vi "main.vi"(0 "Test Pins":T7, 1 "Caller Information":T8, 5 "Test Inputs":T12={"Input Voltage in V"=6.0, "Load Current in A"=[], "Nominal Output Voltage in V"=0.0, "Advance Setting"={"Prepare"={"Load SMU Output Function"=enum."VoltageSource"}, "Stimulus And Measure"={"Loop Delay in milliSecond"=1}}}, 11 "error in":errorcluster) -> (4 "Test Results":T11 {"Load Regulation in mV/mA" format="%#.5g"; "Measured Input Voltage in V" format="%#.5g"; "Measured Input Current in A" format="%#.5g"; "Measured Load Current in A" format="%#.5g"; "Measured Output Voltage in V" format="%#.5g"}, 15 "error out":errorcluster)   [LabVIEW 2020, in "LDO Load Regulation.lvlib"]
doc: "<b>Caller</b> Information is input for framework components. Mode should be set to <b>Automation</b> when running from TestStand. Sequence Context should be set to <b>ThisContext</b> when running from TestStand. The values will be updated everytime the setting is applied using \"Edit\" dialog.\n\n<b>Test Pins</b> is names of pins available in the pinmap file. Provide the right pins for the required functionality.\n\n<b>Test Inputs</b> is input required for the measurement to perform.\n\n<b>error in</b> is meant for the sequencing. <b>error in</b> should be <b>no error</b> always.\n\n<b>Test Results</b> contains all the measured data during the measurement and processed results.\n\n<b>error out</b> contains the error occured during measurement.\n\nCheck measurement documentation for more information (<Program Files>\\Soliton Technologies\\MeasurementSuite\\CodeModules\\LDO\\LDO Load Regulation.pdf)"
uses:
  LDO Load Regulation.lvlib
  Typedefs/Test Results.ctl
  Typedefs/Test Inputs.ctl
  Typedefs/Advance Settings.ctl
  Typedefs/Adv Setup.ctl
  Reusables/Instrument APIs/Load Output Function.ctl
  Typedefs/Adv StimulusMeasure.ctl
  <userlib>/_Soliton/Measurement Suite/Reusables/Plugin Common/Typedefs/Caller Events.ctl
  <userlib>/_Soliton/Measurement Suite/Reusables/Plugin Common/Typedefs/Caller Information.ctl
  <userlib>/_Soliton/Measurement Suite/Reusables/Plugin Common/Typedefs/Caller Mode.ctl
  Typedefs/Test Pins.ctl
  Typedefs/Pin Dropdown.ctl
  <userlib>/_Soliton/Measurement Suite/Reusables/Plugin Common/Typedefs/Termination Monitor Info.ctl
  <vilib>/Utility/error.llb/DialogType.ctl
  dc46d5cc-eb00-4f7e-b59b-e7fbb9f2ed4c.vi
  f0cc231b-6294-4813-9d5b-a7ddc5043ff2.vi
  f8cfc4b9-01f6-4b8f-8ca0-5ef2fe22dc8a.vi
  be024a05-4f6c-4aec-bf2b-5f4e194505bf.vi
  d9360132-6dee-4b9e-876e-39170c807331.vi
  f5d431a0-41a8-4d91-8ed4-f3030fcb2f72.vi
  a0f7aff6-54e5-4632-b7fd-dab2f19ee789.vi
  9bf00ac7-c58e-45e8-95f2-565a27dd0209.vi
  d12a1fd7-5478-4f09-8baf-cc2a5bf82fd5.vi
  97045b22-c088-492e-b8fe-756b4ca626c0.vi
  c2b1c575-6273-4f01-9f2a-bc195d2502fa.vi
  <userlib>/_Soliton/Measurement Suite/Reusables/InstrumentSessionAPIs/SessionManagerApiPath.vi
  <vilib>/Utility/sysdir.llb/Get System Directory.vi
  <vilib>/Utility/LVLibp/Get Exported File Path.vi
  <userlib>/_Soliton/Measurement Suite/Reusables/Errors/Error 6001.vi
  <userlib>/_Soliton/Measurement Suite/Reusables/Plugin Common/Plugin Common.lvlib
  <userlib>/_Soliton/Measurement Suite/Reusables/Queue Driver/Plugin Queue Driver.lvlib
panel:
  out "Progress":i32(slide) scale=-1.0..5.0
  in  "Terminate":bool
  in  "Run":bool caption="Measure"
  in  "Exit":bool
  out "Header":string
  in  "Pages":T1(radio)
  out "Tab Control":T2(tab)
  in  "SystemSetup":T4={"Set Input Voltage"={"PinStatus"=0, "PinName"="", "Info"=TRUE}, "Measure Input Voltage"={"PinStatus"=0, "PinName"="", "Info"=TRUE}, "Measure Input Current"={"PinStatus"=0, "PinName"="", "Info"=TRUE}, "Set Load Current"={"PinStatus"=0, "PinName"="", "Info"=TRUE}, "Measure Output Voltage"={"PinStatus"=0, "PinName"="", "Info"=TRUE}, "Measure Load Current"={"PinStatus"=0, "PinName"="", "Info"=TRUE}}
  in  "Advanced Settings":bool
  in  "Input Voltage (V)":dbl=6.0 format="%#_6p"
  in  "Step Input":T5 {"Step Size (A)" min=0.0 format="%#_6p"; "Stop Value (A)" format="%#_6p"; "Start Value (A)" format="%#_6p"}
  in  "Customize Sweep Value":bool
  in  "Load Current (A)":dbl[](array[numeric]) format="%#_6p"
  in  "Nominal Output Voltage (V)":dbl format="%#_6p"
  in  "Customize Sweep Value":enum32{"Item 0", "Item 1"}(radio)
  out "Load Regulation (mV/mA)":dbl format="%#.3g"
  out "Result Tab":T6(tab)
  out "Line Regulation":cluster{"Iload (mA)":dbl[], "Vout (V)":dbl[]}(graph)
  out "Measured Values":string[][](table)
  out "Load Regulation (%)":dbl format="%#.3g"
  in  "Result Pages":T6(radio)
  in  "DataLogPath":path
  in  "Caller Events":T10
  in  "ErrorOccured":errorcluster
  # "Supports NIDmmInstrument"
  # "Supports NIDmmInstrument"
  # "Supports NIDCPowerInstrument"
  # "Supports NIDCPowerInstrument"
  # "Supports NIDCPowerInstrument"
  # "Supports NIDCPowerInstrument"
  # "Fill Load Current list using the following"
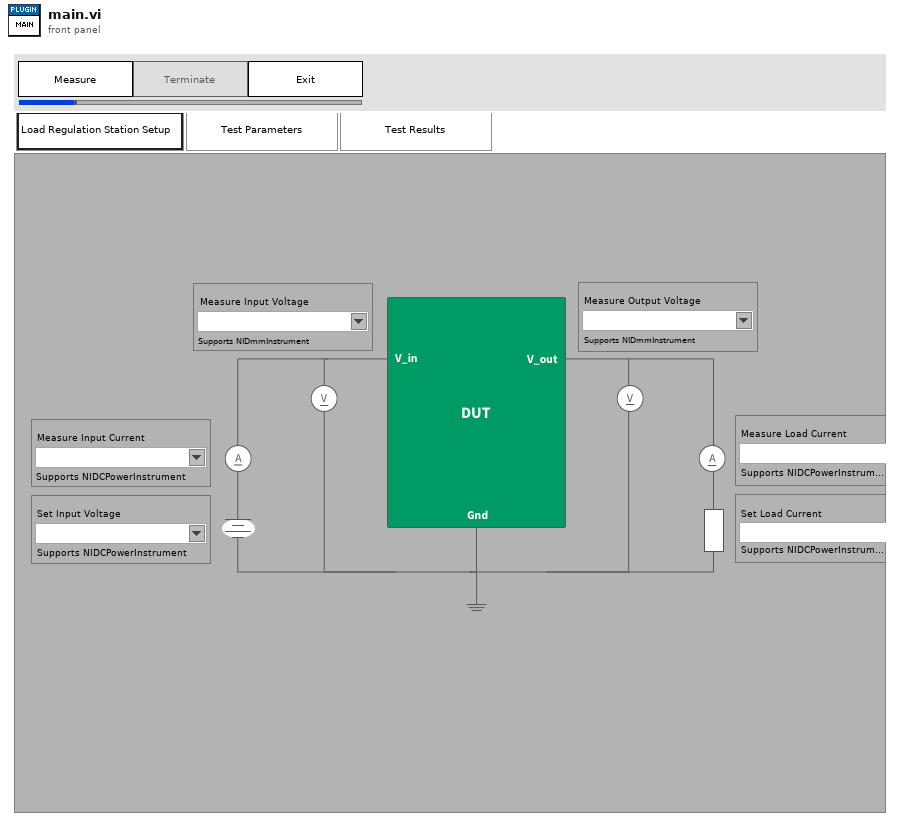
[diagram p1: front panel]
types:
  T1 = enum32{"Station Setup", "Test Parameters", "Test Results"}
  T2 = enum32{"Station Setup", "Test Parameters", "Test Results", "Debug"}
  T3 = typedef "LDO Load Regulation.lvlib/Pin Dropdown.ctl" = cluster{"PinStatus":u16, "PinName":string, "Info":bool}
  T4 = cluster{"Set Input Voltage":T3, "Measure Input Voltage":T3, "Measure Input Current":T3, "Set Load Current":T3, "Measure Output Voltage":T3, "Measure Load Current":T3}
  T5 = cluster{"Start Value (A)":dbl, "Stop Value (A)":dbl, "Step Size (A)":dbl}
  T6 = enum32{"Load Regulation Curve", "Measured Value Table View"}
  T7 = typedef "LDO Load Regulation.lvlib/Test Pins.ctl" = cluster{"Set Input Voltage":string, "Measure Input Voltage":string, "Measure Input Current":string, "Set Load Current":string, "Measure Output Voltage":string, "Measure Load Current":string}
  T8 = typedef "Plugin Common.lvlib/Caller Information.ctl" = cluster{"Mode":T9, "Sequence Context":refnum<k7>}
  T9 = typedef "Caller Mode.ctl" = enum16{"Standalone", "Automation", "MeasurementSuite"}
  T10 = typedef "Plugin Common.lvlib/Caller Events.ctl" = cluster{"Caller Event":refnum<user-event>}
  T11 = typedef "LDO Load Regulation.lvlib/Test Results.ctl" = cluster{"Measured Input Voltage in V":dbl[], "Measured Input Current in A":dbl[], "Measured Output Voltage in V":dbl[], "Measured Load Current in A":dbl[], "Load Regulation in Percentage":dbl, "Load Regulation in mV/mA":dbl}
  T12 = typedef "LDO Load Regulation.lvlib/Test Inputs.ctl" = cluster{"Input Voltage in V":dbl, "Load Current in A":dbl[], "Nominal Output Voltage in V":dbl, "Advance Setting":T13}
  T13 = typedef "LDO Load Regulation.lvlib/Advance Settings.ctl" = cluster{"Prepare":T14, "Stimulus And Measure":T16}
  T14 = typedef "LDO Load Regulation.lvlib/Adv Setup.ctl" = cluster{"Load SMU Output Function":T15}
  T15 = typedef "Load Output Function.ctl" = enum16{"VoltageSource", "CurrentSource"}
  T16 = typedef "LDO Load Regulation.lvlib/Adv StimulusMeasure.ctl" = cluster{"Loop Delay in milliSecond":u32}
  T17 = typedef "Plugin Common.lvlib/Termination Monitor Info.ctl" = cluster{"Caller Information":T8, "Execution":refnum<k7>, "Termination Monitor":refnum<k7>, "Type":string, "Plugin Name":string}
  T18 = cluster{"Termination Monitor Info":T17, "Test Inputs":T12, "Test Results":T11, "Test Results[][]":string[][], "Test Pins":T7, "Logger Folder Path":path, "UI Ctls":refnum<vi>[]}
  T19 = enum8{"Enabled", "Disabled", "Disabled and Grayed Out"}
  T20 = cluster{"Set Vin":T3, "Measure Vin":T3, "Measure Iin":T3, "Set Iload":T3, "Measure Vout":T3, "Measure Iout":T3}
  T21 = cluster{"Start Value":dbl, "Stop Value":dbl, "Step Size":dbl}
  T22 = cluster{"Measured Load Current in A":dbl[], "Measured Output Voltage in V":dbl[]}
  T23 = typedef "DialogType.ctl" = u16
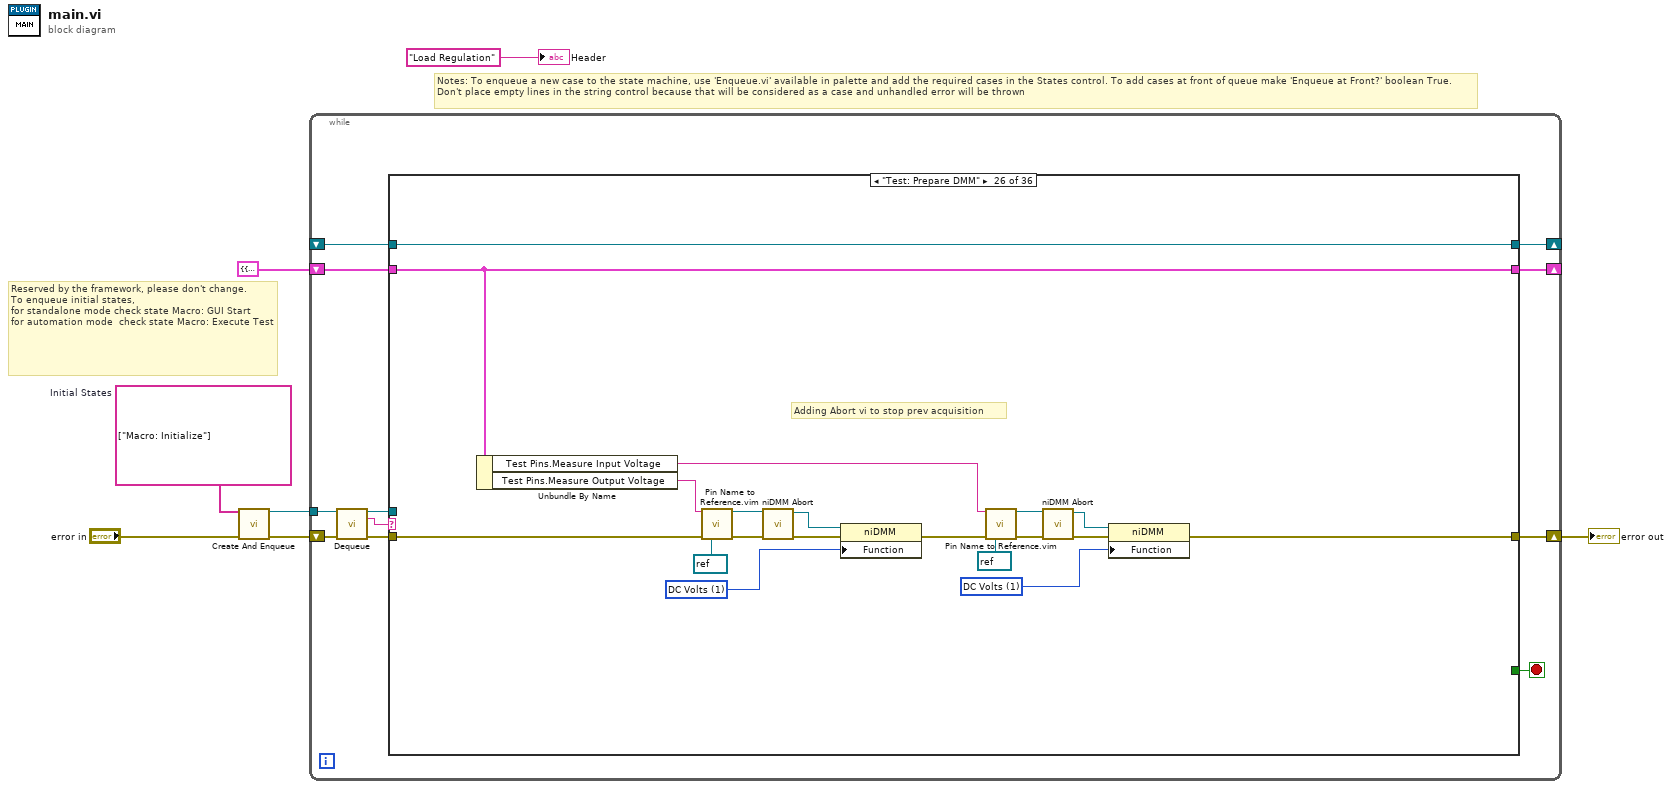
[diagram p0: block diagram]
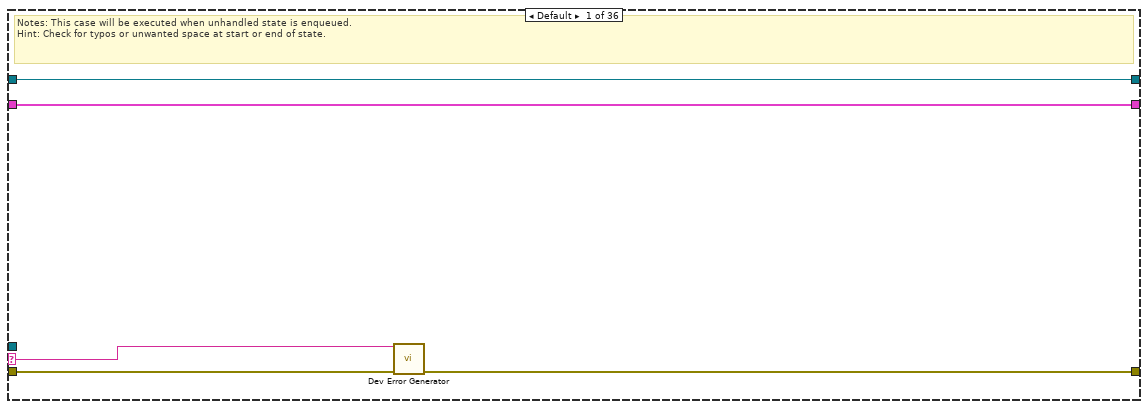
[diagram p2: hidden frame]
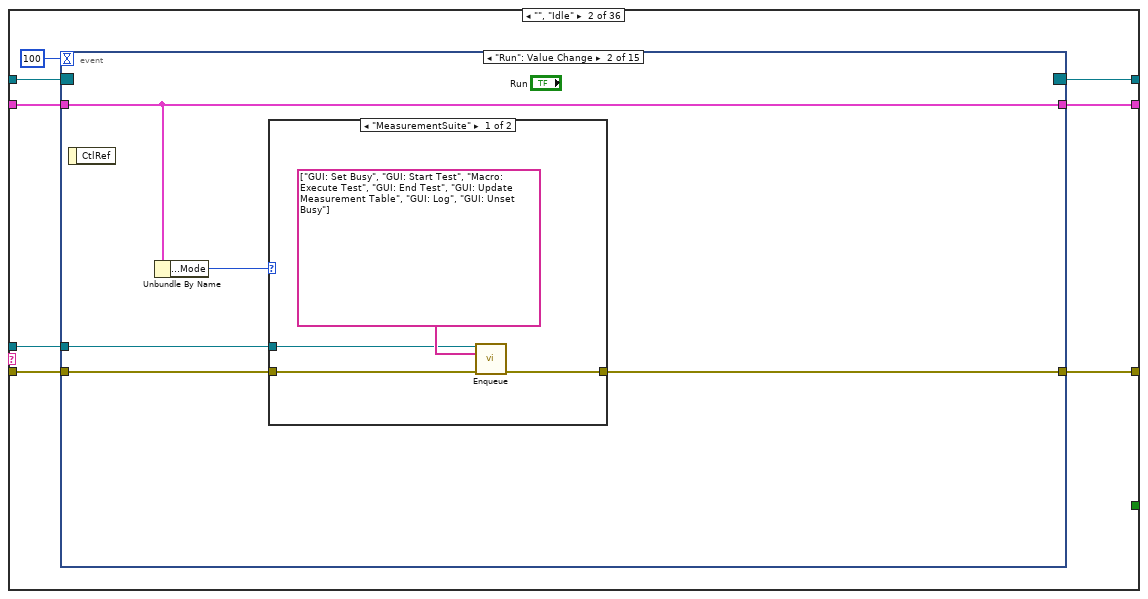
[diagram p3: hidden frame]
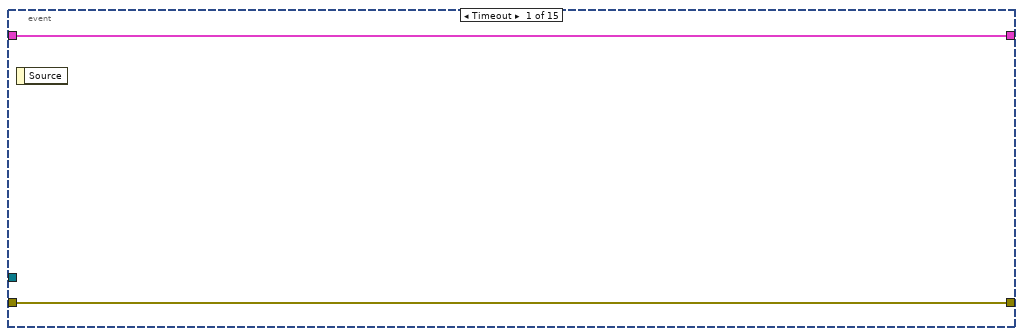
[diagram p4: hidden frame]
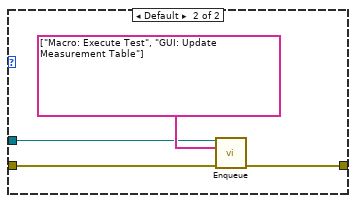
[diagram p5: hidden frame]
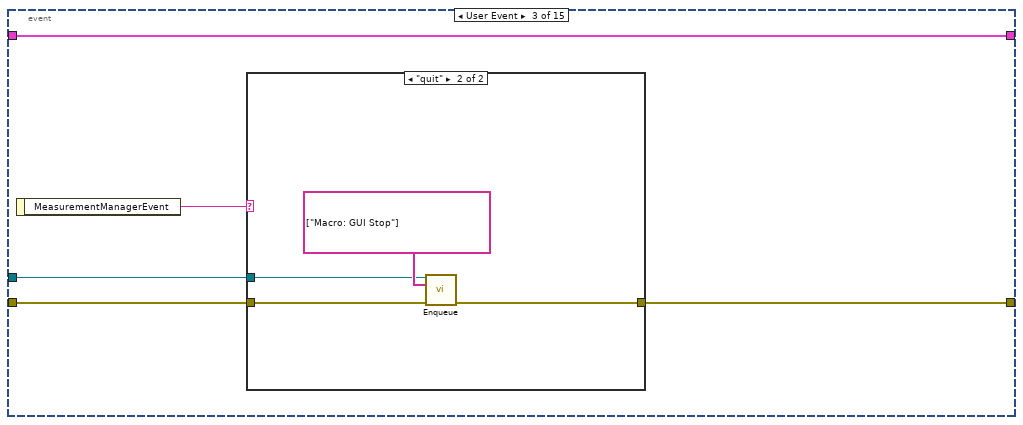
[diagram p6: hidden frame]
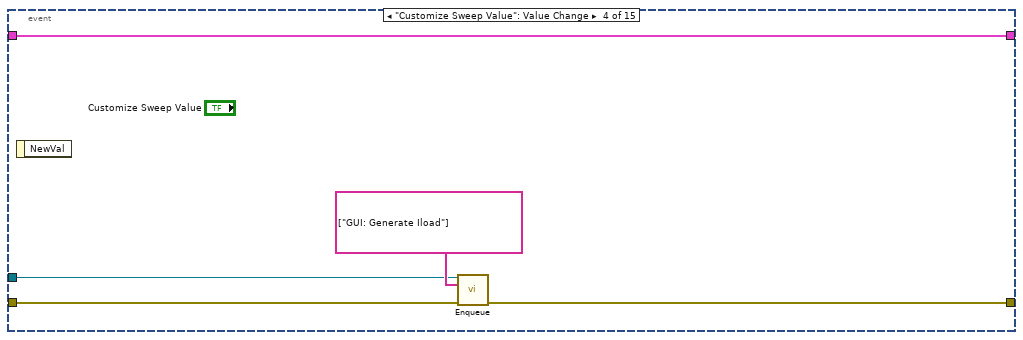
[diagram p8: hidden frame]
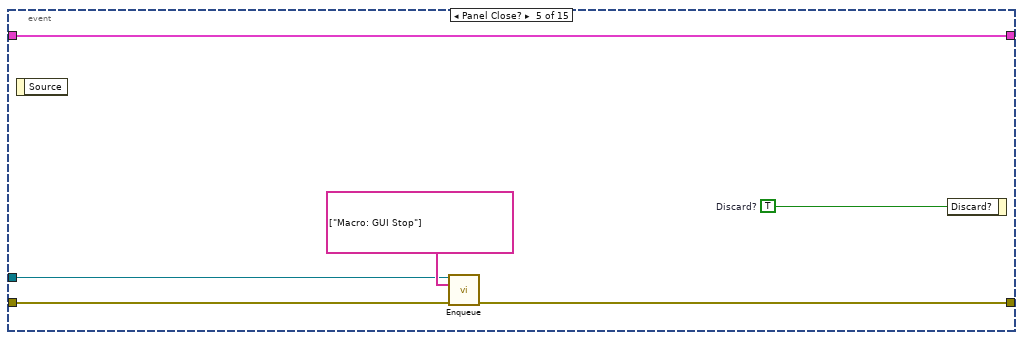
[diagram p9: hidden frame]
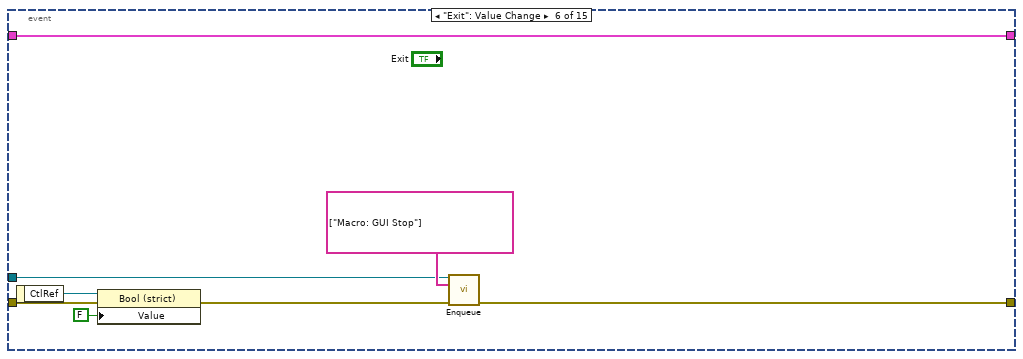
[diagram p10: hidden frame]
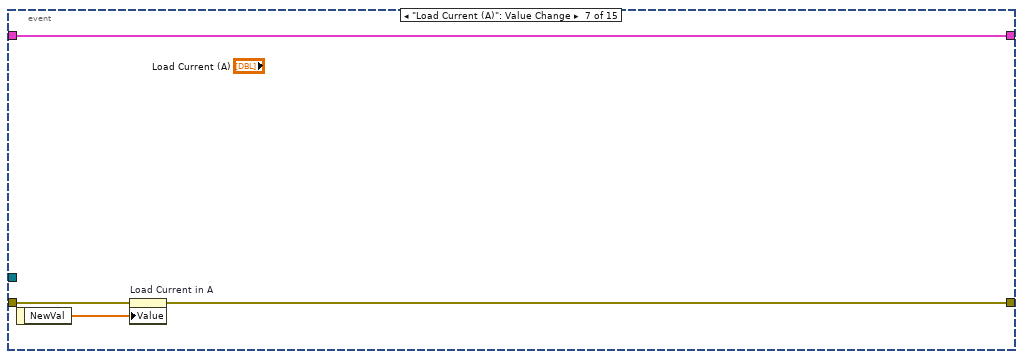
[diagram p11: hidden frame]
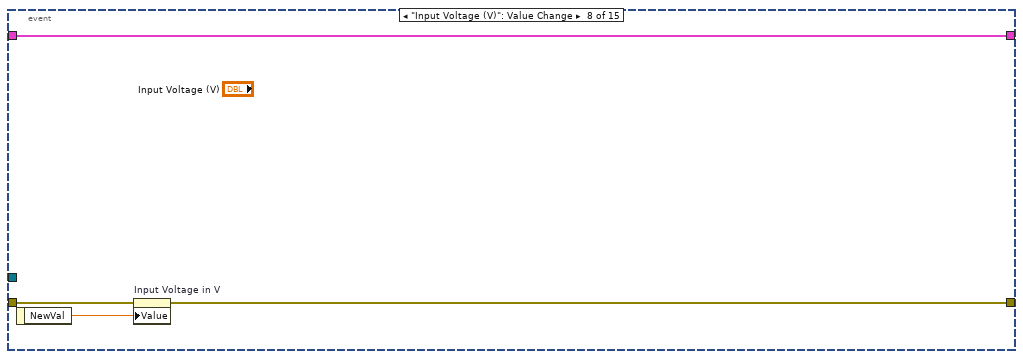
[diagram p12: hidden frame]
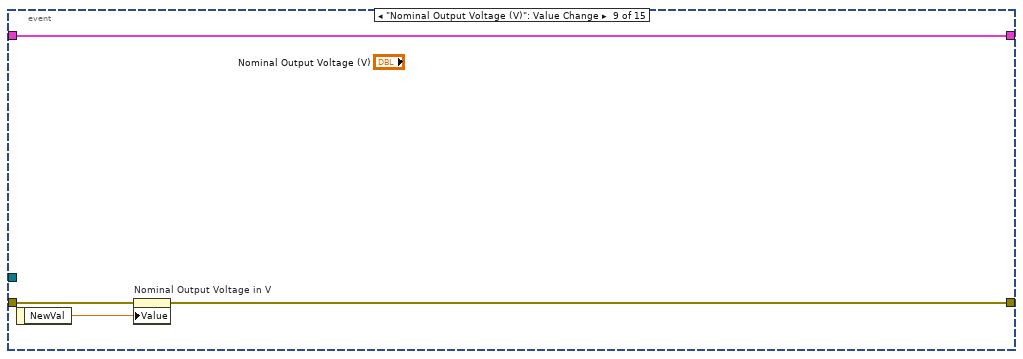
[diagram p13: hidden frame]
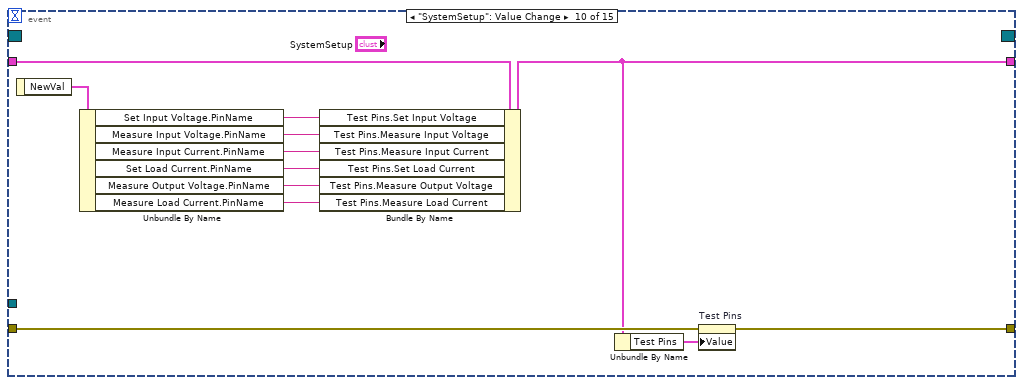
[diagram p14: hidden frame]
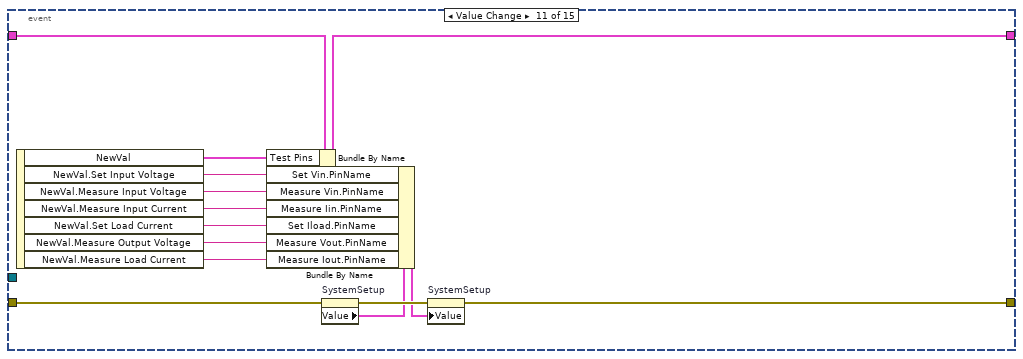
[diagram p15: hidden frame]
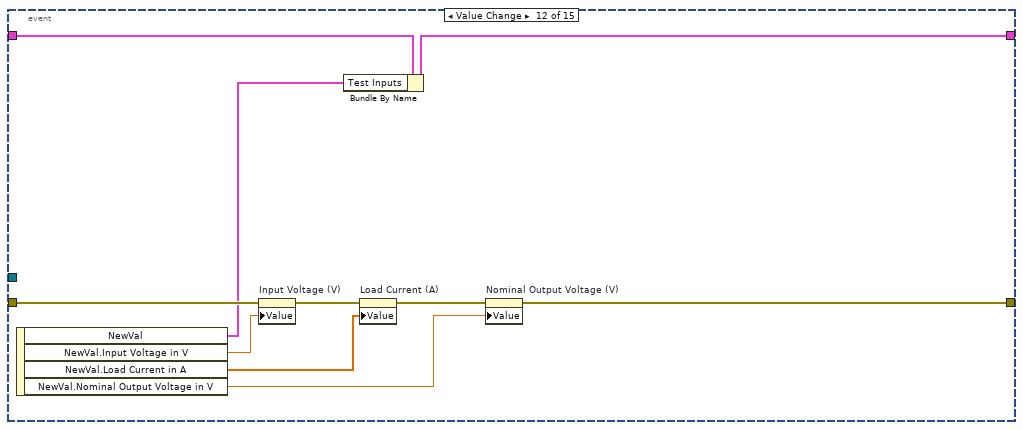
[diagram p16: hidden frame]
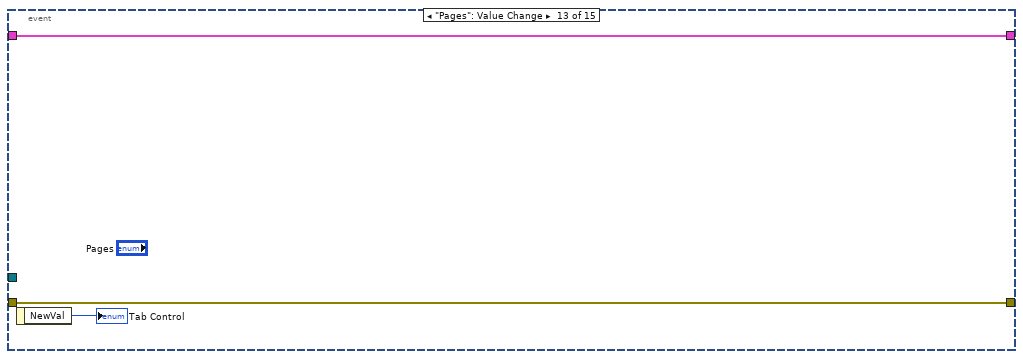
[diagram p17: hidden frame]
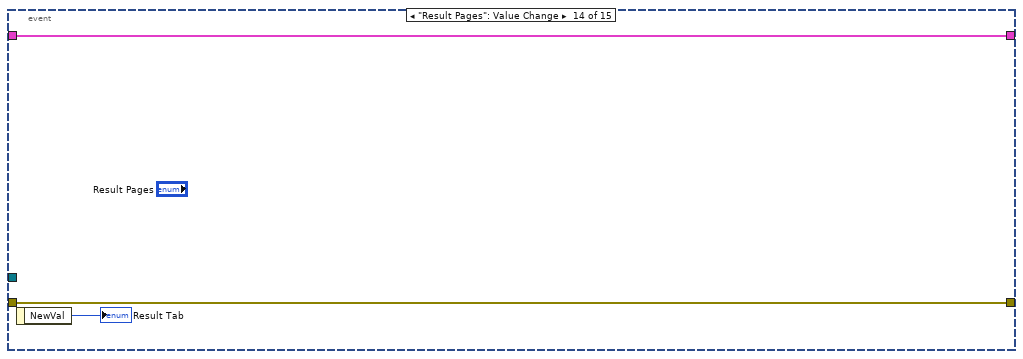
[diagram p18: hidden frame]
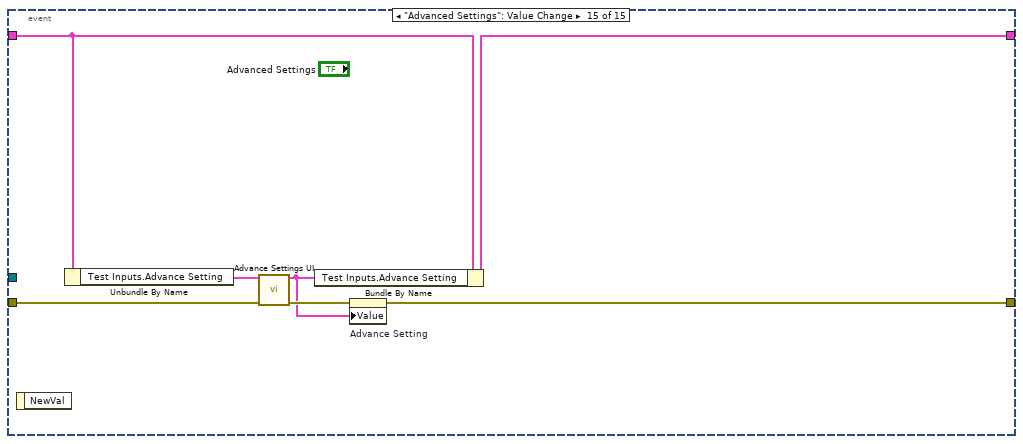
[diagram p19: hidden frame]
diagram:
  w7 = string[] ["Macro: Initialize"]  # Initial States
  # "Notes: To enqueue a new case to the state machine, use 'Enqueue.vi' available in palette and add the required cases in the States control. To add cases at front of queue make 'Enqueue at Front?' boolean True. Don't place empty lines in the string control because that will be considered as a case and unhandled error will be thrown"
  # "Reserved by the framework, please don't change. \nTo enqueue initial states,\nfor standalone mode check state Macro: GUI Start\nfor automation mode  check state Macro: Execute Test"
  n1 = call <userlib>:"Create And Enqueue.vi"("Initial States"=w7, "error in (no error)"="error in") -> ("Queue out"=w5:refnum<queue>, "error out"=w3:errorcluster)  [unwired: 12 in]
  n2 = while {
    shift-right: [w18] -> w4
    shift-left: w3 -> [w16]
    shift-right: [w14] -> _
    shift-left: T18 {"Termination Monitor Info"={"Caller Information"={"Mode"=enum."Standalone", "Sequence Context"=refnum}, "Execution"=refnum, "Termination Monitor"=refnum, "Type"="", "Plugin Name"=""}, "Test Inputs"={"Input Voltage in V"=0.0, "Load Current in A"=[], "Nominal Output Voltage in V"=0.0, "Advance Setting"={"Prepare"={"Load SMU Output Function"=enum."VoltageSource"}, "Stimulus And Measure"={"Loop Delay in milliSecond"=0}}}, "Test Results"={"Measured Input Voltage in V"=[], "Measured Input Current in A"=[], "Measured Output Voltage in V"=[], "Measured Load Current in A"=[], "Load Regulation in Percentage"=0.0, "Load Regulation in mV/mA"=0.0}, "Test Results[][]"=[], "Test Pins"={"Set Input Voltage"="", "Measure Input Voltage"="", "Measure Input Current"="", "Set Load Current"="", "Measure Output Voltage"="", "Measure Load Current"=""}, "Logger Folder Path"=path "", "UI Ctls"=[]} -> [w13]
    tunnel: w5 -> [w12]
    shift-right: [w9] -> _
    shift-left: _ -> [w10]
    stop <- w17 stop-if-true
    n3 = call <userlib>:"Dequeue.vi"("Queue in"=w12, "error in (no error)"=w16) -> ("Queue out"=w11:refnum<queue>, "Dequeued State"=w8:string, "error out"=w15:errorcluster)  [unwired: 11 in]
    n4 = case shown="\"Test: Prepare DMM\"" w8 {
      selector: w8 -> [w21 _ _ _ _ _ _ _ _ _ _ _ _ _ _ _ _ _ _ _ _ _ _ _ _ _ _ _ _ _ _ _ _ _ _ _]
      tunnel: w15 -> [w20 w28 w139 w148 w157 w164 w171 w176 w201 w214 w218 w221 w236 w256 w263 w276 w292 w299 w315 w323 w328 w335 w340 w342 w359 w377 w384 w408 w451 w469 w490 w502 w503 w510 w517 w535]
      tunnel: [w22 w29 w139 w151 w158 w165 w172 w176 w199 w212 w216 w221 w230 w256 w258 w270 w286 w302 w312 w323 w329 w336 w340 w343 w356 w370 w382 w415 w446 w465 w490 w502 w504 w510 w515 w529] -> w18
      tunnel: [_ _ _ _ _ _ _ _ _ _ _ _ _ _ _ _ _ _ _ _ _ _ _ _ _ _ _ _ _ _ _ _ _ _ w512 TRUE] -> w17
      tunnel: [w23 w31 w138 w141 w159 w166 w173 w175 w180 w213 w217 w220 w224 w248 w262 w275 w294 w303 w320 w322 w327 w334 w339 w346 w360 w378 w386 w417 w449 w468 w491 w501 w507 w509 w514 w536] -> w14
      tunnel: w13 -> [w23 w30 w138 w152 w159 w166 w173 w175 w206 w213 w217 w220 w223 w247 w262 w275 w294 w303 w320 w322 w326 w333 w339 w350 w360 w378 w386 w418 w449 w468 w492 w501 w507 w509 w514 w536]
      tunnel: w11 -> [_ w24 _ w150 w155 w162 w169 _ _ _ _ _ _ _ _ _ _ _ _ _ _ _ _ _ _ _ _ _ _ _ _ _ _ _ w511 w534]
      tunnel: w10 -> [w19 w26 w137 w149 w154 w161 w168 w174 w205 _ w215 w219 w237 w255 w265 w278 w293 w304 w319 w321 w330 w337 w338 w348 w361 w380 w385 w416 w463 w476 w493 w500 w506 w508 w516 w533]
      tunnel: [w19 w25 w137 w149 w154 w161 w168 w174 w205 w211 w215 w219 w237 w255 w265 w278 w293 w304 w319 w321 w330 w337 w338 w348 w361 w380 w385 w416 w463 w476 w493 w500 w506 w508 w516 w533] -> w9
      frame Default {
        # "Notes: This case will be executed when unhandled state is enqueued. \nHint: Check for typos or unwanted space at start or end of state."
        n5 = call <userlib>:"Dev Error Generator.vi"("State"=w21, "error in (no error)"=w20) -> ("error out"=w22:errorcluster)  [unwired: 13 in]
      }
      frame "", "Idle" {
        n6 = event shown="[1] \"Run\": Value Change" {
          selector: w26 -> [_ _ _ _ _ _ _ _ _ _ _ _ _ _ _]
          dyn-events: [_ _ _ _ _ _ _ _ _ _ _ _ _ _ _] -> w25
          timeout: 100 -> [_ _ _ _ _ _ _ _ _ _ _ _ _ _ _]
          tunnel: [w33 w35 w51 w61 w67 w75 w76 w83 w87 w89 w108 w116 w126 w129 w131] -> w31
          tunnel: w30 -> [w33 w35 w51 w61 w67 w75 w76 w83 w87 w93 w107 w115 w126 w129 w130]
          tunnel: [w32 w38 w49 w59 w64 w73 w78 w82 w86 w91 w111 w118 w125 w128 w134] -> w29
          tunnel: w28 -> [w32 w37 w50 w58 w63 w72 w79 w81 w85 w90 w113 w123 w125 w128 w135]
          tunnel: w24 -> [_ w36 w47 w57 w62 w71 _ _ _ _ _ _ _ _ _]
          event Timeout {
            n7 = event-data() -> ()  [unwired: 1 in, 1 out]
          }
          event "Run": Value Change {
            n8 = event-data() -> ()  [unwired: 1 in, 1 out]
            n9 = Unbundle By Name(w35) -> ("Termination Monitor Info.Caller Information.Mode"=w34:T9)
            n10 = case shown="\"MeasurementSuite\"" w34 {
              tunnel: [w41 w45] -> w38
              tunnel: w37 -> [w40 w44]
              tunnel: w36 -> [w39 w43]
              frame "MeasurementSuite" {
                n11 = call <userlib>:"Enqueue.vi"("Queue in"=w39, "States"=string[] ["GUI: Set Busy", "GUI: Start Test", "Macro: Execute Test", "GUI: End Test", "GUI: Update Measurement Table", "GUI: Log", "GUI: Unset Busy"], "error in (no error)"=w40) -> ("error out"=w41:errorcluster)  [unwired: 11 in, 1 out]
              }
              frame Default {
                n12 = call <userlib>:"Enqueue.vi"("Queue in"=w43, "States"=string[] ["Macro: Execute Test", "GUI: Update Measurement Table"], "error in (no error)"=w44) -> ("error out"=w45:errorcluster)  [unwired: 11 in, 1 out]
              }
            }
          }
          event User Event {
            n13 = event-data() -> ("MeasurementManagerEvent"=w48:string)  [unwired: 1 in]
            n14 = case shown="\"quit\"" w48 {
              tunnel: [w52 w53] -> w49
              tunnel: w50 -> [w52 w55]
              tunnel: w47 -> [_ w54]
              frame Default {
              }
              frame "quit" {
                n15 = call <userlib>:"Enqueue.vi"("Queue in"=w54, "States"=string[] ["Macro: GUI Stop"], "error in (no error)"=w55) -> ("error out"=w53:errorcluster)  [unwired: 11 in, 1 out]
              }
            }
          }
          event "Customize Sweep Value": Value Change {
            n16 = event-data() -> ()  [unwired: 1 in, 1 out]
            n17 = call <userlib>:"Enqueue.vi"("Queue in"=w57, "States"=string[] ["GUI: Generate Iload"], "error in (no error)"=w58) -> ("error out"=w59:errorcluster)  [unwired: 11 in, 1 out]
          }
          event Panel Close? {
            w66 = TRUE  # Discard?
            n18 = event-data() -> ()  [unwired: 1 in, 1 out]
            n19 = call <userlib>:"Enqueue.vi"("Queue in"=w62, "States"=string[] ["Macro: GUI Stop"], "error in (no error)"=w63) -> ("error out"=w64:errorcluster)  [unwired: 11 in, 1 out]
            n20 = event-data("Discard?"=w66) -> ()  [unwired: 1 in, 1 out]
          }
          event "Exit": Value Change {
            n21 = event-data() -> ("CtlRef"=w69:refnum<vi>)  [unwired: 1 in]
            n22 = property class="Bool (strict)"(reference=w69, error in=w72, "Value"=FALSE) -> (error out=w70:errorcluster)  [unwired: 1 out]
            n23 = call <userlib>:"Enqueue.vi"("Queue in"=w71, "States"=string[] ["Macro: GUI Stop"], "error in (no error)"=w70) -> ("error out"=w73:errorcluster)  [unwired: 11 in, 1 out]
          }
          event "Load Current (A)": Value Change {
            n24 = event-data() -> ("NewVal"=w77:dbl[])  [unwired: 1 in]
            n25 = property on="Load Current in A" class="Arr (strict)"(error in=w79, "Value"=w77) -> (error out=w78:errorcluster)  [unwired: 1 in, 1 out]
          }
          event "Input Voltage (V)": Value Change {
            n26 = event-data() -> ("NewVal"=w80:dbl)  [unwired: 1 in]
            n27 = property on="Input Voltage in V" class="DigNum (strict)"(error in=w81, "Value"=w80) -> (error out=w82:errorcluster)  [unwired: 1 in, 1 out]
          }
          event "Nominal Output Voltage (V)": Value Change {
            n28 = event-data() -> ("NewVal"=w84:dbl)  [unwired: 1 in]
            n29 = property on="Nominal Output Voltage in V" class="DigNum (strict)"(error in=w85, "Value"=w84) -> (error out=w86:errorcluster)  [unwired: 1 in, 1 out]
          }
          event "SystemSetup": Value Change {
            n30 = event-data() -> ("NewVal"=w92:T4)  [unwired: 1 in]
            n31 = Unbundle By Name(w92) -> ("Set Input Voltage.PinName"=w99:string, "Measure Input Voltage.PinName"=w98:string, "Measure Input Current.PinName"=w97:string, "Set Load Current.PinName"=w96:string, "Measure Output Voltage.PinName"=w95:string, "Measure Load Current.PinName"=w94:string)
            n32 = Bundle By Name(cluster=w93, "Test Pins.Set Input Voltage"=w99, "Test Pins.Measure Input Voltage"=w98, "Test Pins.Measure Input Current"=w97, "Test Pins.Set Load Current"=w96, "Test Pins.Measure Output Voltage"=w95, "Test Pins.Measure Load Current"=w94) -> (w89:T18)
            n33 = Unbundle By Name(w89) -> ("Test Pins"=w88:T7)
            n34 = property on="Test Pins" class="Clust (strict)"(error in=w90, "Value"=w88) -> (error out=w91:errorcluster)  [unwired: 1 in, 1 out]
          }
          event Value Change {
            n35 = event-data() -> ("NewVal"=w100:T7, "NewVal.Set Input Voltage"=w106:string, "NewVal.Measure Input Voltage"=w105:string, "NewVal.Measure Input Current"=w104:string, "NewVal.Set Load Current"=w103:string, "NewVal.Measure Output Voltage"=w102:string, "NewVal.Measure Load Current"=w101:string)  [unwired: 1 in]
            n36 = Bundle By Name(cluster=w107, "Test Pins"=w100) -> (w108:T18)
            n37 = property on="SystemSetup" class="Clust (strict)"(error in=w113) -> (error out=w112:errorcluster, "Value"=w110:T20)  [unwired: 1 in, 1 out]
            n38 = Bundle By Name(cluster=w110, "Set Vin.PinName"=w106, "Measure Vin.PinName"=w105, "Measure Iin.PinName"=w104, "Set Iload.PinName"=w103, "Measure Vout.PinName"=w102, "Measure Iout.PinName"=w101) -> (w109:T20)
            n39 = property on="SystemSetup" class="Clust (strict)"(error in=w112, "Value"=w109) -> (error out=w111:errorcluster)  [unwired: 1 in, 1 out]
          }
          event Value Change {
            n40 = event-data() -> ("NewVal"=w114:T12, "NewVal.Input Voltage in V"=w120:dbl, "NewVal.Load Current in A"=w119:dbl[], "NewVal.Nominal Output Voltage in V"=w117:dbl)  [unwired: 1 in]
            n41 = property on="Input Voltage (V)" class="DigNum (strict)"(error in=w123, "Value"=w120) -> (error out=w122:errorcluster)  [unwired: 1 in, 1 out]
            n42 = Bundle By Name(cluster=w115, "Test Inputs"=w114) -> (w116:T18)
            n43 = property on="Load Current (A)" class="Arr (strict)"(error in=w122, "Value"=w119) -> (error out=w121:errorcluster)  [unwired: 1 in, 1 out]
            n44 = property on="Nominal Output Voltage (V)" class="DigNum (strict)"(error in=w121, "Value"=w117) -> (error out=w118:errorcluster)  [unwired: 1 in, 1 out]
          }
          event "Pages": Value Change {
            n45 = event-data() -> ("NewVal"=→"Tab Control":T1)  [unwired: 1 in]
          }
          event "Result Pages": Value Change {
            n46 = event-data() -> ("NewVal"=→"Result Tab":T6)  [unwired: 1 in]
          }
          event "Advanced Settings": Value Change {
            n47 = event-data() -> ()  [unwired: 1 in, 1 out]
            n48 = Unbundle By Name(w130) -> ("Test Inputs.Advance Setting"=w133:T13)
            n49 = call "Advance Settings UI.vi"("Advance Setting"=w133, "error in (no error)"=w135) -> ("Advance Setting Out"=w132:T13, "error out"=w136:errorcluster)  [unwired: 12 in]
            n50 = Bundle By Name(cluster=w130, "Test Inputs.Advance Setting"=w132) -> (w131:T18)
            n51 = property on="Advance Setting" class="Clust (strict)"(error in=w136, "Value"=w132) -> (error out=w134:errorcluster)  [unwired: 1 in, 1 out]
          }
        }
      }
      frame "----------------- Macro ---------------" {
        # "Not used. category splitter"
      }
      frame "Macro: Initialize" {
        w145 = string[] ["Macro: GUI Start"]  # Standalone: Start the debug
        w146 = string[] ["Macro: Execute Test", "Exit"]  # Automation: Execute and stop
        # "Hidden in UI"
        # "This case decides the mode of the execution. Debug Mode: The plugin will act as a standalone GUI where user can change inputs, run test and debug the system. automation mode: The plugin will act as a flat code and go through all the test procedures and stops."
        n52 = call <userlib>:"Get Mode.vi"("Caller Information"="Caller Information", "error in (no error)"=w148) -> ("Automation(F) \\ Standalone (T)"=w144:bool, "error out"=w147:errorcluster)  [unwired: 12 in]
        n53 = Bundle By Name(cluster=w152, "Termination Monitor Info.Caller Information"="Caller Information") -> (w141:T18)
        n54 = Select(t=w145, s=w144, f=w146) -> (s? t:f=w143:string[])
        n55 = call <userlib>:"Enqueue.vi"("Queue in"=w150, "States"=w143, "Enqueue at Front?(F)"=TRUE, "error in (no error)"=w147) -> ("error out"=w151:errorcluster)  [unwired: 10 in, 1 out]
      }
      frame "Macro: Execute Test" {
        w156 = string[] ["TerminationMonitor: Start", "Test: Start", "Test: Prepare DCPower", "Test: Prepare DMM", "Test: Set Input Voltage", "Test: Sweep Over Load", "Test: Cleanup DCPower", "Test: Cleanup DMM", "Test: Calculate Load", "Test: Update UI", "Test: End", "TerminationMonitor: Stop"]  # Test Procedure
        # "List the states required for the test procedure. This state will be called in both automation mode and standalone mode when requested to run the test.\nDont remove 'Test: Start' and 'Test: End'."
        n56 = call <userlib>:"Enqueue.vi"("Queue in"=w155, "States"=w156, "Enqueue at Front?(F)"=TRUE, "error in (no error)"=w157) -> ("error out"=w158:errorcluster)  [unwired: 10 in, 1 out]
      }
      frame "Macro: GUI Start" {
        # "Initialize the data cluster for the standalone mode and register for the event from caller.\nDon't remove 'GUI: Initialize Data' and 'GUI: Register Event'."
        n57 = call <userlib>:"Enqueue.vi"("Queue in"=w162, "States"=string[] ["GUI: Initialize Data", "GUI: Register Event"], "Enqueue at Front?(F)"=TRUE, "error in (no error)"=w164) -> ("error out"=w165:errorcluster)  [unwired: 10 in, 1 out]
      }
      frame "Macro: GUI Stop" {
        # "Cleanups the standalone mode and stop the execution.\nDon't remove 'GUI: Unregister Event', 'GUI: Cleanup Data' and 'Exit'."
        n58 = call <userlib>:"Enqueue.vi"("Queue in"=w169, "States"=string[] ["GUI: Unregister Event", "GUI: Cleanup Data", "Exit"], "Enqueue at Front?(F)"=TRUE, "error in (no error)"=w171) -> ("error out"=w172:errorcluster)  [unwired: 10 in, 1 out]
      }
      frame "--------------- GUI Mode-----------------" {
        # "Not used. category splitter"
      }
      frame "GUI: Initialize Data" {
        w194 = T6."Load Regulation Curve" ("Result Enum")
        w193 = T1."Station Setup" ("Tab Enum")
        w197 = string[][] []  # Test Results[][]
        w208 = T11 {"Measured Input Voltage in V"=[], "Measured Input Current in A"=[], "Measured Output Voltage in V"=[], "Measured Load Current in A"=[], "Load Regulation in Percentage"=0.0, "Load Regulation in mV/mA"=0.0}  # Test Results
        # "Add the front panel controls terminal here and connect them to the bundle structure, So they will be available through data cluster in every case. If the controls and indicators are added to the 'Test Inputs' & 'Test Results' cluster then they are already available in the data cluster since they are typedefs."
        n59 = property on="Run" class="Bool (strict)"(error in=w201, "DisabledEnum"=T19."Enabled" ("Disabled")) -> (error out=w204:errorcluster)  [unwired: 1 in, 1 out]
        n60 = property on="Terminate" class="Bool (strict)"(error in=w204, "DisabledEnum"=T19."Disabled and Grayed Out" ("Disabled")) -> (error out=w200:errorcluster)  [unwired: 1 in, 1 out]
        n61 = Bundle By Name(cluster=w206, "Test Pins"="Test Pins", "Test Inputs"="Test Inputs", "Test Results"=w208, "Test Results[][]"=w197, "Logger Folder Path"="DataLogPath") -> (w207:T18)
        n62 = property on="Progress" class="Slide (strict)"(error in=w200, "Visible"=FALSE) -> (error out=w199:errorcluster)  [unwired: 1 in, 1 out]
        n63 = control-ref of="Customize Sweep Value"() -> (w185:refnum<vi>)
        n64 = control-ref of="Pages"() -> (w182:refnum<vi>)
        n65 = control-ref of="Result Pages"() -> (w181:refnum<vi>)
        n66 = control-ref of="Customize Sweep Value"() -> (w186:refnum<vi>)
        n67 = control-ref of="Advanced Settings"() -> (w184:refnum<vi>)
        n68 = control-ref of="SystemSetup"() -> (w178:refnum<vi>)
        n69 = control-ref of="Load Regulation (mV/mA)"() -> (w177:refnum<vi>)
        n70 = control-ref of="Input Voltage (V)"() -> (w192:refnum<vi>)
        n71 = control-ref of="Nominal Output Voltage (V)"() -> (w191:refnum<vi>)
        n72 = control-ref of="Start Value (A)"() -> (w189:refnum<vi>)
        n73 = control-ref of="Stop Value (A)"() -> (w188:refnum<vi>)
        n74 = control-ref of="Step Size (A)"() -> (w187:refnum<vi>)
        n75 = control-ref of="Load Regulation (%)"() -> (w183:refnum<vi>)
        n76 = control-ref of="Load Current (A)"() -> (w190:refnum<vi>)
        n77 = Build Array(w192, w191, w190, w189, w188, w187, w186, w185, w184, w183, w182, w181, w178, w177) -> (w179:refnum<vi>[])
        n78 = Bundle By Name(cluster=w207, "UI Ctls"=w179) -> (w180:T18)
        n79 = local write "Tab Control"(w193) -> ()
        n80 = local write "Result Pages"(w194) -> ()
        n81 = local write "Result Tab"(w194) -> ()
        n82 = local write "Pages"(w193) -> ()
      }
      frame "GUI: Register Event" {
        # "Hidden in UI"
        # "Register for the events from caller."
        n83 = register-events(error in=w214, "Caller Events") -> (reference out=w211:refnum<event-registration>, error out=w212:errorcluster)  [unwired: 1 in]
      }
      frame "GUI: Unregister Event" {
        n84 = Unregister For Events(event registration refnum=w215, error in=w218) -> (error out=w216:errorcluster)
      }
      frame "GUI: Cleanup Data" {
        # "Cleanup the reference or other resources before exiting"
      }
      frame "GUI: Generate Iload" {
        n85 = property on="Step Input" class="Clust (strict)"(error in=w236) -> (error out=w225:errorcluster, "Value"=w235:T21)  [unwired: 1 in, 1 out]
        n86 = Unbundle By Name(w235) -> ("Start Value"=w234:dbl, "Stop Value"=w233:dbl, "Step Size"=w232:dbl)
        n87 = property on="Customize Sweep Value" class="RadioBtnsControl (strict)"(error in=w225) -> (error out=w227:errorcluster, "Value"=w229:enum32{"Item 0", "Item 1"})  [unwired: 1 in, 1 out]
        n88 = call "Get Range Values[].vi"("Start"=w234, "Stop"=w233, "Step Size"=w232) -> ("Values[]"=w228:dbl[])  [unwired: 12 in]
        n89 = case shown="\"Item 1\"" w229 {
          tunnel: w228 -> [w239 w240]
          tunnel: [w239 w242] -> w222
          tunnel: w227 -> [w238 w244]
          tunnel: [w238 w243] -> w226
          frame "Item 0", Default {
          }
          frame "Item 1" {
            # "Append to end"
            n90 = property on="Load Current (A)" class="Arr (strict)"(error in=w244) -> (error out=w243:errorcluster, "Value"=w241:dbl[])  [unwired: 1 in, 1 out]
            n91 = Insert Into Array(array=w241, new element=w240) -> (w242:dbl[])  [unwired: 1 in]
          }
        }
        n92 = property on="Load Current (A)" class="Arr (strict)"(error in=w226, "Value"=w222) -> (error out=w231:errorcluster)  [unwired: 1 in, 1 out]
        n93 = Bundle By Name(cluster=w223, "Test Inputs.Load Current in A"=w222) -> (w224:T18)
        n94 = property on="Load Current in A" class="Arr (strict)"(error in=w231, "Value"=w222) -> (error out=w230:errorcluster)  [unwired: 1 in, 1 out]
      }
      frame "GUI: Update Measurement Table" {
        n95 = Unbundle By Name(w247) -> ("Test Results.Measured Input Voltage in V"=w254:dbl[], "Test Results.Measured Input Current in A"=w253:dbl[], "Test Results.Measured Output Voltage in V"=w251:dbl[], "Test Results.Measured Load Current in A"=w250:dbl[])
        n96 = Build Array(w254, w253, w251, w250) -> (w252:dbl[][])
        n97 = Transpose 2D Array(2D array=w252) -> (transposed array=w249:dbl[][])
        n98 = Number To Fractional String(number=w249, precision (6)=i16 5) -> (F-format string=w246:string[][])  [unwired: 2 in]
        "Measured Values" <- w246
        n99 = Bundle By Name(cluster=w247, "Test Results[][]"=w246) -> (w248:T18)
      }
      frame "GUI: Set Busy" {
        n100 = Unbundle By Name(w262) -> ("UI Ctls"=w261:refnum<vi>[])
        n101 = for {
          tunnel: [w268] -> w264 mode=indexing
          tunnel: w263 -> [w269]
          tunnel: w261 -> [w267] mode=indexing
          tunnel: T19."Disabled and Grayed Out" ("Disabled") -> [w266]
          n102 = property class="Ctl"(reference=w267, error in=w269, "DisabledEnum"=w266) -> (error out=w268:errorcluster)  [unwired: 1 out]
        }
        n103 = Merge Errors(w264) -> (w259:errorcluster)
        n104 = call "Defer Front Panel.vi"("Defer Front Panel?"=TRUE, "error in"=w259) -> ("error out"=w258:errorcluster)  [unwired: 13 in]
      }
      frame "GUI: Unset Busy" {
        n105 = Unbundle By Name(w275) -> ("UI Ctls"=w274:refnum<vi>[])
        n106 = for {
          tunnel: [w281] -> w277 mode=indexing
          tunnel: w276 -> [w282]
          tunnel: w274 -> [w280] mode=indexing
          tunnel: T19."Enabled" ("Disabled") -> [w279]
          n107 = property class="Ctl"(reference=w280, error in=w282, "DisabledEnum"=w279) -> (error out=w281:errorcluster)  [unwired: 1 out]
        }
        n108 = Merge Errors(w277) -> (w271:errorcluster)
        n109 = call "Defer Front Panel.vi"("Defer Front Panel?"=FALSE, "error in"=w271) -> ("error out"=w270:errorcluster)  [unwired: 13 in]
      }
      frame "GUI: Start Test" {
        n110 = property on="Run" class="Bool (strict)"(error in=w292, "DisabledEnum"=T19."Disabled and Grayed Out" ("Disabled")) -> (error out=w290:errorcluster)  [unwired: 1 in, 1 out]
        n111 = property on="Terminate" class="Bool (strict)"(error in=w290, "DisabledEnum"=T19."Enabled" ("Disabled")) -> (error out=w287:errorcluster)  [unwired: 1 in, 1 out]
        n112 = Unbundle By Name(w294) -> ("Test Inputs.Load Current in A"=w285:dbl[])
        n113 = Array Size(array=w285) -> (size(s)=w284:i32)
        n114 = property on="Progress" class="Slide (strict)"(error in=w287, "Visible"=TRUE, "Scale.Maximum"=w284, "Value"=0 ("Progress")) -> (error out=w286:errorcluster)  [unwired: 1 in, 1 out]
      }
      frame "GUI: Log" {
        n115 = Unbundle By Name(w303) -> ("Test Inputs"=w300:T12, "Test Results"=w301:T11, "Logger Folder Path"=w297:path)
        n116 = call <vilib>:"Check if File or Folder Exists.vi"("error in (no error)"=w299, "path"=w297) -> ("error out"=w298:errorcluster, "file or folder exists?"=w295:bool, "dup path"=w296:path)  [unwired: 7 in]
        n117 = case shown="True" w295 {
          tunnel: [w305 w310] -> w302
          tunnel: w298 -> [w305 w309]
          tunnel: w301 -> [_ w308]
          tunnel: w300 -> [_ w307]
          tunnel: w296 -> [_ w306]
          frame False {
          }
          frame True {
            n118 = call "Log Data.vi"("Test Inputs"=w307, "Test Results"=w308, "DataLogger File Path"=w306, "error in (no error)"=w309) -> ("error out"=w310:errorcluster)  [unwired: 11 in]
          }
        }
      }
      frame "GUI: End Test" {
        n119 = property on="Run" class="Bool (strict)"(error in=w315, "Value"=FALSE ("Run"), "DisabledEnum"=T19."Enabled" ("Disabled")) -> (error out=w318:errorcluster)  [unwired: 1 in, 1 out]
        n120 = property on="Terminate" class="Bool (strict)"(error in=w318, "DisabledEnum"=T19."Disabled and Grayed Out" ("Disabled")) -> (error out=w313:errorcluster)  [unwired: 1 in, 1 out]
        n121 = property on="Progress" class="Slide (strict)"(error in=w313, "Visible"=FALSE) -> (error out=w312:errorcluster)  [unwired: 1 in, 1 out]
      }
      frame "------------ TerminationMonitor -----------" {
        # "Not used. category splitter"
      }
      frame "TerminationMonitor: Start" {
        # "Termination Monitor monitors the execution of the caller. Use Termination Monitor Status to get the termination status. If the caller is terminating, stop the test procedure, cleanup and stop."
        n122 = Unbundle By Name(w326) -> ("Termination Monitor Info.Caller Information"=w325:T8)
        n123 = call <userlib>:"Termination Monitor Start.vi"("Caller Information"=w325, "error in (no error)"=w328) -> ("Termination Monitor Info out"=w324:T17, "error out"=w329:errorcluster)  [unwired: 12 in]
        n124 = Bundle By Name(cluster=w326, "Termination Monitor Info"=w324) -> (w327:T18)
      }
      frame "TerminationMonitor: Stop" {
        n125 = Unbundle By Name(w333) -> ("Termination Monitor Info"=w332:T17)
        n126 = call <userlib>:"Termination Monitor Stop.vi"("Status Info in"=w332, "error in (no error)"=w335) -> ("Status Info out"=w331:T17, "error out"=w336:errorcluster)  [unwired: 12 in]
        n127 = Bundle By Name(cluster=w333, "Termination Monitor Info"=w331) -> (w334:T18)
      }
      frame "------------ Automation Mode -----------" {
        # "Not used. category splitter"
      }
      frame "Test: Start" {
        # "Reinitialize/Reset/Update the data from the UI to the data cluster so that the data will be considered for the test procedure.\nReset the Test Results."
        n128 = property on="Progress" class="Slide (strict)"(error in=w342, "Value"=0 ("Progress")) -> (error out=w343:errorcluster)  [unwired: 1 in, 1 out]
        n129 = local read "DataLogPath"() -> (w344:path)
        n130 = local read "Test Inputs"() -> (w349:T12)
        n131 = local read "Test Pins"() -> (w345:T7)
        n132 = Bundle By Name(cluster=w350, "Test Pins"=w345, "Test Inputs"=w349, "Test Results"=T11 {"Measured Input Voltage in V"=[], "Measured Input Current in A"=[], "Measured Output Voltage in V"=[], "Measured Load Current in A"=[], "Load Regulation in Percentage"=0.0, "Load Regulation in mV/mA"=0.0}, "Logger Folder Path"=w344) -> (w346:T18)
      }
      frame "Test: Prepare DCPower" {
        # "Set Input voltage as initial voltage level\nSet first index of Load current as initial current"
        n133 = Unbundle By Name(w360) -> ("Test Pins.Set Load Current"=w358:string, "Test Inputs.Load Current in A"=w354:dbl[], "Test Inputs.Advance Setting.Prepare.Load SMU Output Function"=w355:T15, "Test Pins.Set Input Voltage"=w353:string, "Test Inputs.Input Voltage in V"=w352:dbl)
        n134 = call "Prepare Source.vi"("Set Vin"=w353, "Initial Voltage Level (V)"=w352, "error in (no error)"=w359) -> ("error out"=w357:errorcluster)  [unwired: 12 in]
        n135 = Index Array(array=w354) -> (element=w351:dbl)  [unwired: 1 in]
        n136 = call "Prepare Load.vi"("PinName"=w358, "Load Current Level (A)"=w351, "error in (no error)"=w357, "Load Output Function"=w355) -> ("error out"=w356:errorcluster)  [unwired: 11 in]
      }
      frame "Test: Prepare DMM" {
        w374 = 1 items=["DC Volts"=1, "AC Volts"=2, "DC Current"=3, "AC Current"=4, "2-Wire Resistance"=5, "4-Wire Resistance"=101, "Frequency"=104, "Period"=105, "AC Volts DC Coupled"=1001, "Diode"=1002, "Waveform Voltage"=1003, "Waveform Current"=1004, "Capacitance"=1005, "Inductance"=1006, "Temperature"=108] ("Configuration:Function")
        w375 = 1 items=["DC Volts"=1, "AC Volts"=2, "DC Current"=3, "AC Current"=4, "2-Wire Resistance"=5, "4-Wire Resistance"=101, "Frequency"=104, "Period"=105, "AC Volts DC Coupled"=1001, "Diode"=1002, "Waveform Voltage"=1003, "Waveform Current"=1004, "Capacitance"=1005, "Inductance"=1006, "Temperature"=108] ("Configuration:Function")
        # "Adding Abort vi to stop prev acquisition"
        n137 = Unbundle By Name(w378) -> ("Test Pins.Measure Input Voltage"=w368:string, "Test Pins.Measure Output Voltage"=w369:string)
        n138 = call "Pin Name to Reference.vim"("Pin Name"=w369, "type"=refnum<k15> refnum ("instrument handle"), "error in (no error)"=w377) -> ("Reference"=w366:refnum<k15>, "error out"=w376:errorcluster)  [unwired: 7 in, 4 out]
        n139 = call <instrlib>:"niDMM Abort.vi"("error in (no error)"=w376, "instrument handle"=w366) -> ("error out"=w367:errorcluster, "instrument handle out"=w365:refnum<k15>)  [unwired: 8 in]
        n140 = property class="niDMM"(reference=w365, error in=w367, "Function"=w375) -> (error out=w371:errorcluster)  [unwired: 1 out]
        n141 = call "Pin Name to Reference.vim"("Pin Name"=w368, "type"=refnum<k15> refnum ("instrument handle"), "error in (no error)"=w371) -> ("Reference"=w363:refnum<k15>, "error out"=w373:errorcluster)  [unwired: 7 in, 4 out]
        n142 = call <instrlib>:"niDMM Abort.vi"("error in (no error)"=w373, "instrument handle"=w363) -> ("error out"=w364:errorcluster, "instrument handle out"=w362:refnum<k15>)  [unwired: 8 in]
        n143 = property class="niDMM"(reference=w362, error in=w364, "Function"=w374) -> (error out=w370:errorcluster)  [unwired: 1 out]
      }
      frame "Test: Set Input Voltage" {
        # "Do any sort of programming\\feel free to be innovative and make sure you document the code for the yourself and other engineers benefits. Split the procedure into different modular cases."
        n144 = Unbundle By Name(w386) -> ("Test Pins.Set Input Voltage"=w383:string, "Test Inputs.Input Voltage in V"=w381:dbl)
        n145 = call "Set Source.vi"("Set Vin"=w383, "Vin in V"=w381, "error in (no error)"=w384) -> ("error out"=w382:errorcluster)  [unwired: 12 in]
      }
      frame "Test: Sweep Over Load" {
        n146 = Unbundle By Name(w418) -> ("Termination Monitor Info"=w414:T17, "Test Inputs.Advance Setting.Stimulus And Measure.Loop Delay in milliSecond"=w390:u32, "Test Pins.Set Load Current"=w392:string, "Test Inputs.Load Current in A"=w389:dbl[], "Test Inputs.Advance Setting.Prepare.Load SMU Output Function"=w387:T15, "Test Pins.Measure Input Current"=w398:string, "Test Pins.Measure Load Current"=w399:string, "Test Pins.Measure Input Voltage"=w400:string, "Test Pins.Measure Output Voltage"=w401:string)
        n147 = call "Pin Name to Reference.vim"("Pin Name"=w401, "type"=refnum<k15> refnum ("instrument handle"), "error in (no error)"=w408) -> ("Reference"=w394:refnum<k15>, "error out"=w404:errorcluster)  [unwired: 7 in, 4 out]
        n148 = call "Pin Name to Reference.vim"("Pin Name"=w400, "type"=refnum<k15> refnum ("instrument handle"), "error in (no error)"=w404) -> ("Reference"=w395:refnum<k15>, "error out"=w403:errorcluster)  [unwired: 7 in, 4 out]
        n149 = call "Pin Name to Reference.vim"("Pin Name"=w399, "type"=refnum<k15> refnum ("instrument handle"), "error in (no error)"=w403) -> ("Reference"=w396:refnum<k15>, "error out"=w402:errorcluster)  [unwired: 7 in, 4 out]
        n150 = call "Pin Name to Reference.vim"("Pin Name"=w398, "type"=refnum<k15> refnum ("instrument handle"), "error in (no error)"=w402) -> ("Reference"=w397:refnum<k15>, "error out"=w388:errorcluster)  [unwired: 7 in, 4 out]
        n151 = for {
          shift-right: [w444] -> w415
          shift-left: w388 -> [w425]
          shift-right: [w442] -> w393
          shift-left: w414 -> [w443]
          tunnel: [w432] -> w413 mode=indexing
          tunnel: [w431] -> w410 mode=indexing
          tunnel: [w433] -> w412 mode=indexing
          tunnel: [w434] -> w411 mode=indexing
          tunnel: w392 -> [w424]
          tunnel: w397 -> [w438]
          tunnel: w396 -> [w437]
          tunnel: w395 -> [w436]
          tunnel: w394 -> [w435]
          tunnel: w390 -> [w419]
          tunnel: w389 -> [w423] mode=indexing
          tunnel: w387 -> [w422]
          i -> [w440]
          stop <- w441 stop-if-true
          n152 = call "Set Load Current.vi"("PinName"=w424, "current level"=w423, "error in (no error)"=w425, "OutputFunction"=w422) -> ("error out"=w421:errorcluster)  [unwired: 11 in]
          n153 = call "Stall Data Flow.vim"("value in"=w421, "milliseconds to wait"=w419) -> ("value out"=w420:errorcluster)  [unwired: 1 out]
          n154 = call <instrlib>:"niDCPower Measure Multiple.vi"("error in (no error)"=w420, "instrument handle"=w438) -> ("error out"=w427:errorcluster, "current measurements"=w430:dbl[])  [unwired: 6 in, 2 out]
          n155 = Index Array(array=w430) -> (element=w434:dbl)  [unwired: 1 in]
          n156 = call <instrlib>:"niDCPower Measure Multiple.vi"("error in (no error)"=w427, "instrument handle"=w437) -> ("error out"=w426:errorcluster, "current measurements"=w428:dbl[])  [unwired: 6 in, 2 out]
          n157 = Index Array(array=w428) -> (element=w433:dbl)  [unwired: 1 in]
          n158 = call <instrlib>:"niDMM Read.vi"("error in (no error)"=w426, "instrument handle"=w436) -> ("error out"=w429:errorcluster, "Measurement"=w431:dbl)  [unwired: 7 in, 1 out]
          n159 = call <instrlib>:"niDMM Read.vi"("error in (no error)"=w429, "instrument handle"=w435) -> ("error out"=w439:errorcluster, "Measurement"=w432:dbl)  [unwired: 7 in, 1 out]
          n160 = call <userlib>:"Termination Monitor Status.vi"("Termination Monitor Info in"=w443, "error in (no error)"=w439) -> ("Termination Monitor Info out"=w442:T17, "Terminating?"=w441:bool, "error out"=w444:errorcluster)  [unwired: 11 in]
          "Progress" <- w440
        }
        n161 = Negate(x=w412) -> (-x=w391:dbl[])
        n162 = Bundle By Name(cluster=w418, "Termination Monitor Info"=w393, "Test Results.Measured Input Current in A"=w411, "Test Results.Measured Load Current in A"=w391, "Test Results.Measured Input Voltage in V"=w410, "Test Results.Measured Output Voltage in V"=w413) -> (w417:T18)
      }
      frame "Test: Cleanup DCPower" {
        n163 = Unbundle By Name(w449) -> ("Test Pins.Set Input Voltage"=w459:string, "Test Pins.Set Load Current"=w461:string)
        n164 = call "Pin Name to Reference.vim"("Pin Name"=w461, "type"=refnum<k15> refnum ("instrument handle"), "error in (no error)"=w451) -> ("Reference"=w454:refnum<k15>, "error out"=w453:errorcluster)  [unwired: 7 in, 4 out]
        n165 = call <instrlib>:"niDCPower Configure Output Enabled.vi"("error in (no error)"=w453, "output enabled"=FALSE, "instrument handle"=w454) -> ("error out"=w452:errorcluster, "instrument handle out"=w447:refnum<k15>)  [unwired: 7 in]
        n166 = call <instrlib>:"niDCPower Abort With Channels.vi"("error in (no error)"=w452, "instrument handle"=w447) -> ("error out"=w448:errorcluster)  [unwired: 8 in, 1 out]
        n167 = call "Pin Name to Reference.vim"("Pin Name"=w459, "type"=refnum<k15> refnum ("instrument handle"), "error in (no error)"=w448) -> ("Reference"=w456:refnum<k15>, "error out"=w455:errorcluster)  [unwired: 7 in, 4 out]
        n168 = call <instrlib>:"niDCPower Configure Output Enabled.vi"("error in (no error)"=w455, "output enabled"=FALSE, "instrument handle"=w456) -> ("error out"=w450:errorcluster, "instrument handle out"=w445:refnum<k15>)  [unwired: 7 in]
        n169 = call <instrlib>:"niDCPower Abort With Channels.vi"("error in (no error)"=w450, "instrument handle"=w445) -> ("error out"=w446:errorcluster)  [unwired: 8 in, 1 out]
      }
      frame "Test: Cleanup DMM" {
        n170 = Unbundle By Name(w468) -> ("Test Pins.Measure Input Voltage"=w472:string, "Test Pins.Measure Output Voltage"=w474:string)
        n171 = call "Pin Name to Reference.vim"("Pin Name"=w474, "type"=refnum<k15> refnum ("instrument handle"), "error in (no error)"=w469) -> ("Reference"=w466:refnum<k15>, "error out"=w470:errorcluster)  [unwired: 7 in, 4 out]
        n172 = call <instrlib>:"niDMM Abort.vi"("error in (no error)"=w470, "instrument handle"=w466) -> ("error out"=w467:errorcluster)  [unwired: 8 in, 1 out]
        n173 = call "Pin Name to Reference.vim"("Pin Name"=w472, "type"=refnum<k15> refnum ("instrument handle"), "error in (no error)"=w467) -> ("Reference"=w464:refnum<k15>, "error out"=w471:errorcluster)  [unwired: 7 in, 4 out]
        n174 = call <instrlib>:"niDMM Abort.vi"("error in (no error)"=w471, "instrument handle"=w464) -> ("error out"=w465:errorcluster)  [unwired: 8 in, 1 out]
      }
      frame "Test: Calculate Load" {
        n175 = Unbundle By Name(w492) -> ("Test Results.Measured Output Voltage in V"=w486:dbl[], "Test Inputs.Nominal Output Voltage in V"=w484:dbl, "Test Results.Measured Load Current in A"=w481:dbl[])
        n176 = Array Max & Min(array=w486) -> (max value=w489:dbl, min value=w485:dbl)  [unwired: 2 out]
        n177 = Array Max & Min(array=w481) -> (max value=w482:dbl, min value=w483:dbl)  [unwired: 2 out]
        n178 = Subtract(x=w489, y=w485) -> (x-y=w480:dbl)
        n179 = Subtract(x=w482, y=w483) -> (x-y=w479:dbl)
        n180 = Divide(x=w480, y=w479) -> (x/y=w478:dbl)
        n181 = Divide(x=w480, y=w484) -> (x/y=w488:dbl)
        n182 = Multiply(x=w488, y=100.0) -> (x*y=w487:dbl)
        n183 = Bundle By Name(cluster=w492, "Test Results.Load Regulation in Percentage"=w487, "Test Results.Load Regulation in mV/mA"=w478) -> (w491:T18)
      }
      frame "Test: Update UI" {
        # "If you want to update more indicators in the front panel do it here. It is efficient to update the UI in one case rather than in several cases. Also, it is a good practice to store the results in the data cluster in an efficient format and then get the data from data cluster and update the UI, in that way we could have the front panel independent of how we manipulate the data."
        n184 = Unbundle By Name(w501) -> ("Test Results.Measured Load Current in A"=w499:dbl[], "Test Results"=w498:T11, "Test Results.Load Regulation in Percentage"=→"Load Regulation (%)":dbl, "Test Results.Load Regulation in mV/mA"=→"Load Regulation (mV/mA)":dbl)
        "Test Results" <- w498
        n185 = Unbundle By Name(w498) -> ("Measured Output Voltage in V"=w497:dbl[])
        n186 = Bundle("Measured Load Current in A"=w499, "Measured Output Voltage in V"=w497) -> (→"Line Regulation":T22)  [unwired: 1 in]
      }
      frame "Test: End" {
        # "End of the Test Procedure. Do cleanup of resources or references."
        n187 = property on="Progress" class="Slide (strict)"(error in=w503, "Value"=0 ("Progress")) -> (error out=w504:errorcluster)  [unwired: 1 in, 1 out]
      }
      frame "---------------------Misc-----------------------" {
      }
      frame "Error" {
        # "Handle the error and make sure to clear the error."
        n188 = Unbundle By Name(w514) -> ("Termination Monitor Info.Caller Information.Mode"=w513:T9)
        n189 = case shown="\"MeasurementSuite\"" w513 {
          tunnel: w517 -> [w521 w526 w528]
          tunnel: [w519 w523 w527] -> w515
          tunnel: [_ TRUE _] -> w512
          tunnel: w511 -> [_ w524 _]
          frame "Standalone" {
            w518 = T23 2 items=["no dialog", "OK message", "continue or stop message", "OK message + warnings", "continue/stop + warnings"] ("type of dialog (OK msg:1)")
            n190 = call <vilib>:"General Error Handler.vi"("type of dialog (OK msg:1)"=w518, "error in (no error)"=w521) -> ("error out"=w520:errorcluster)  [unwired: 9 in, 4 out]
            n191 = call <vilib>:"Clear Errors.vi"("error in (no error)"=w520) -> ("error out"=w519:errorcluster)  [unwired: 5 in, 1 out]
          }
          frame "Automation" {
            n192 = call <userlib>:"Release.vi"("Queue in"=w524) -> ("Error Out"=w522:errorcluster)  [unwired: 14 in]
            n193 = Merge Errors(w526, w522) -> (w523:errorcluster)
          }
          frame "MeasurementSuite" {
            n194 = property on="ErrorOccured" class="Clust (strict)"("Val(Sgnl)"=w528) -> (error out=w527:errorcluster)  [unwired: 2 in, 1 out]
          }
        }
      }
      frame "Exit" {
        # "Last case called before stopping the execution. \nError occured in this state will not be captured by Error state."
        n195 = call <userlib>:"Release.vi"("Queue in"=w534, "Error In"=w535) -> ("Error Out"=w530:errorcluster)  [unwired: 13 in]
        n196 = property on="Progress" class="Slide (strict)"(error in=w530, "Visible"=TRUE) -> (error out=w529:errorcluster)  [unwired: 1 in, 1 out]
      }
    }
  }
  "error out" <- w4
  "Header" <- "Load Regulation" ("Header")
